vi "数据查询.vi"() -> ()   [LabVIEW 2014]
uses:
  <vilib>/Analysis/baseanly.llb/Mean (DBL).vi
  <vilib>/Analysis/NI_AALBase.lvlib
panel:
  out "平均温度: 2":dbl caption="平均温度:"
  out "最低温度: 2":dbl caption="最低温度:"
  out "最高温度: 2":dbl caption="最高温度:"
  in  "返回":bool
  in  "导出报表":bool
  in  "高级查询":bool
  in  "查询":bool
  in  "查询结果":i32(listbox)
  in  "结束时间：":timestamp format="%<%y/%m/%d>T"
  in  "开始时间：":timestamp format="%<%y/%m/%d>T"
  out "平均温度:":dbl
  out "最低温度:":dbl
  out "最高温度:":dbl
  out "温度":cluster{sgl, sgl}[](graph)
  # "数据查询起止时间设置"
  # "采集参数"
  # "进口温度"
  # "出口温度"
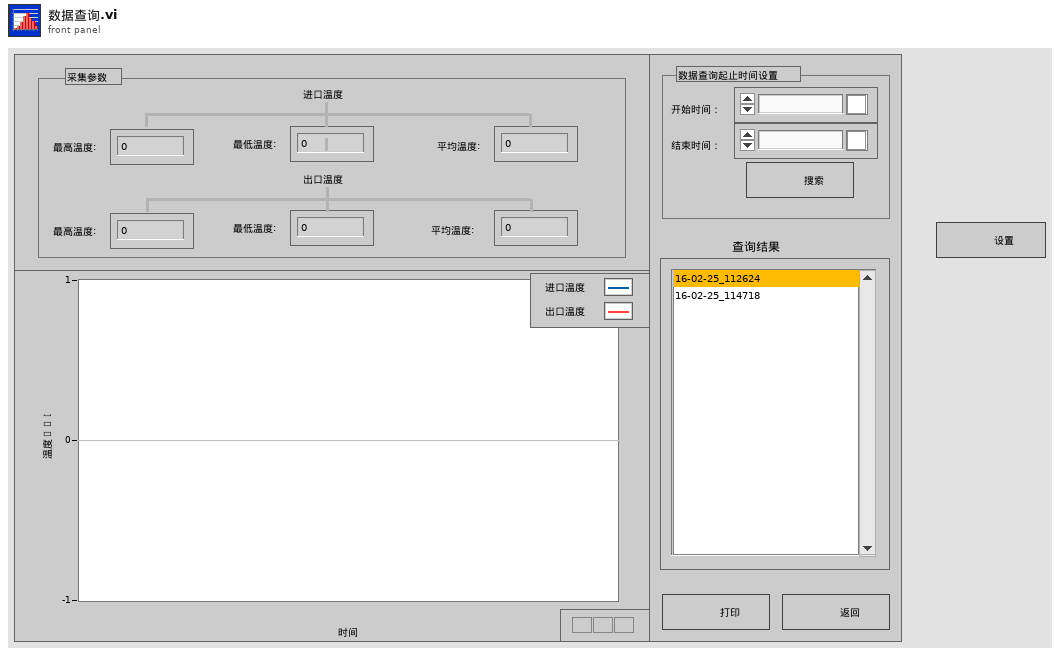
[diagram p1: front panel]
types:
  T1 = enum16{"open", "open or create", "create or replace", "create", "open (read-only)"}
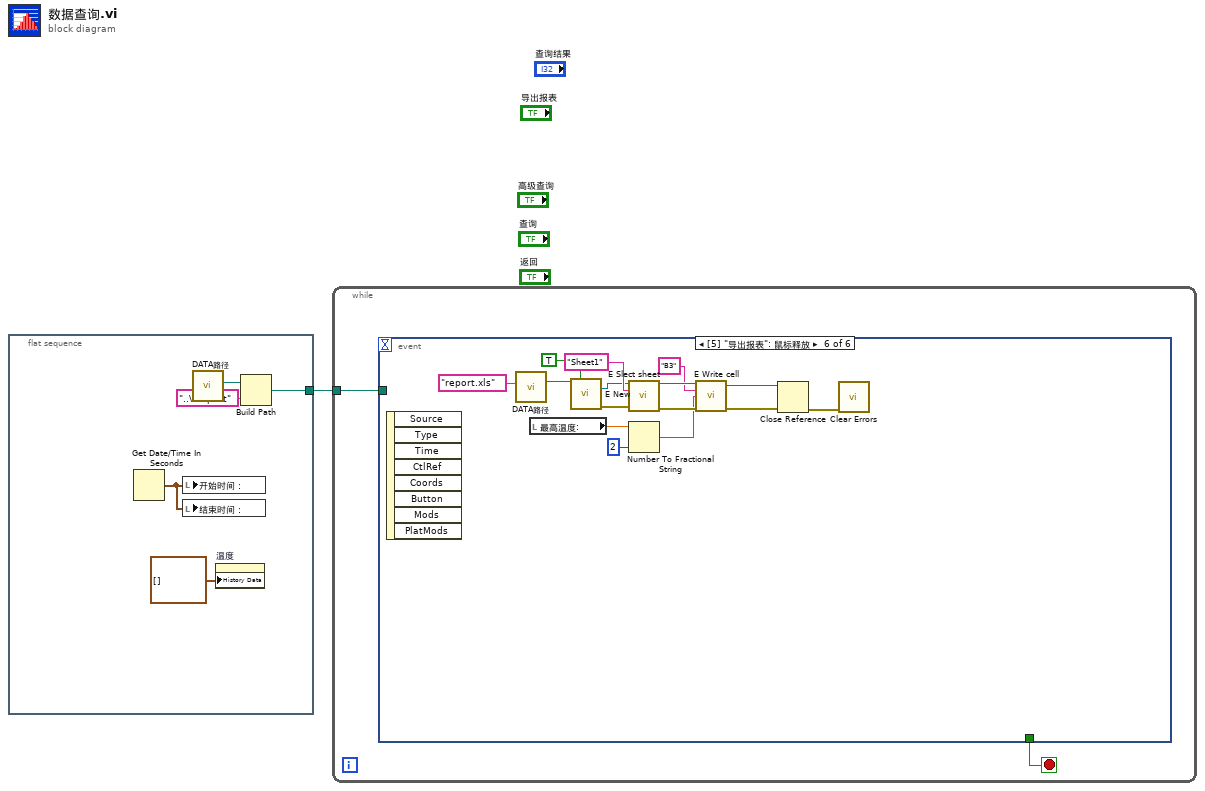
[diagram p0: block diagram]
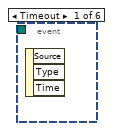
[diagram p2: hidden frame]
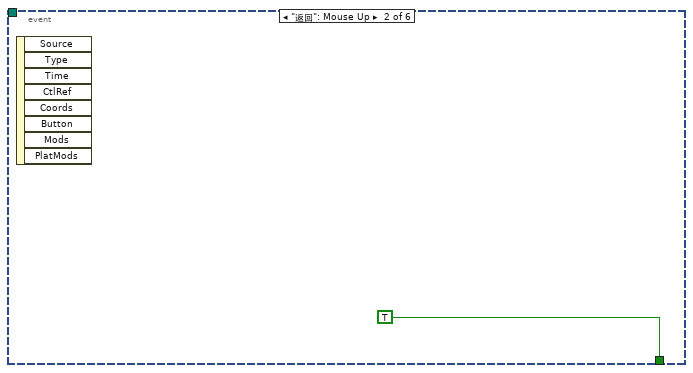
[diagram p3: hidden frame]
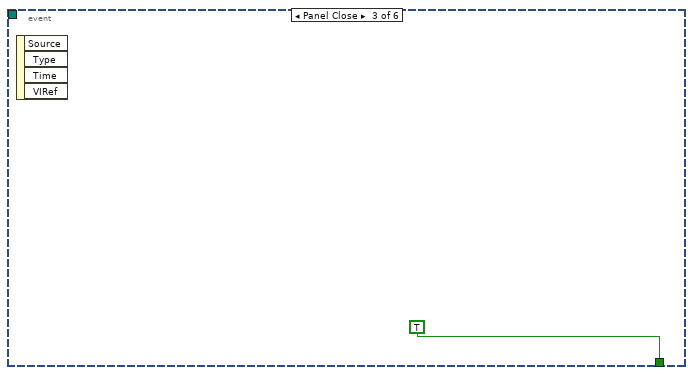
[diagram p4: hidden frame]
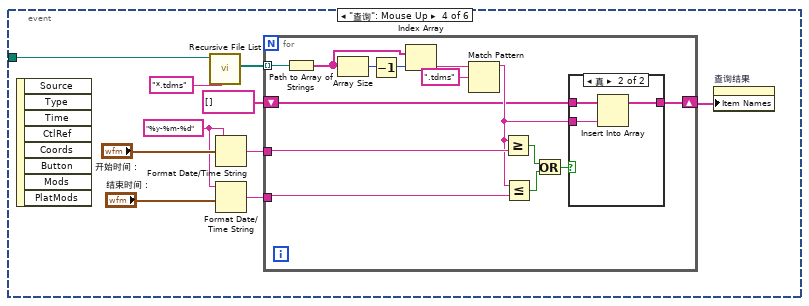
[diagram p5: hidden frame]
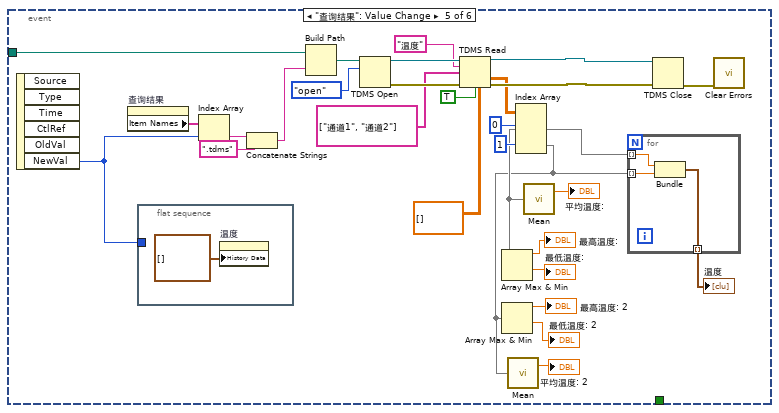
[diagram p7: hidden frame]
diagram:
  n1 = flat-sequence {
    tunnel: [w4] -> w1
    frame #0 {
      n2 = Get Date/Time In Seconds() -> (seconds since 1Jan1904=w3:timestamp)
      n3 = local write "开始时间："(w3) -> ()
      n4 = local write "结束时间："(w3) -> ()
      n5 = call "DATA路径.vi"() -> ("DATA路径"=w6:path)  [unwired: 11 in]
      n6 = property on="温度" class="WFChart (严格)"("History Data"=cluster{sgl, sgl}[] [] ("历史数据")) -> ()  [unwired: 2 in, 2 out]
      n7 = Build Path(base path=w6, name or relative path="..\\Report" ("名称或相对路径")) -> (appended path=w4:path)
    }
  }
  n8 = while {
    tunnel: w1 -> [w7]
    stop <- w8 stop-if-true
    n9 = event shown="[5] \"导出报表\": 鼠标释放" {
      selector: _ -> [_ _ _ _ _ _]
      dyn-events: _ -> [_ _ _ _ _ _]
      timeout: _ -> [_ _ _ _ _ _]
      tunnel: [_ TRUE TRUE _ _ _] -> w8
      tunnel: w7 -> [_ _ _ w17 w66 _]
      event Timeout {
        n10 = event-data() -> ()  [unwired: 1 in, 3 out]
      }
      event "返回": Mouse Up {
        n11 = event-data() -> ()  [unwired: 1 in, 8 out]
      }
      event Panel Close {
        n12 = event-data() -> ()  [unwired: 1 in, 4 out]
      }
      event "查询": Mouse Up {
        w18 = "%y-%m-%d" ("时间格式字符串(%c)")
        n13 = event-data() -> ()  [unwired: 1 in, 8 out]
        n14 = call <vilib>:"Recursive File List.vi"("pattern"="*.tdms", "Folder Path"=w17) -> ("All Files in Dir"=w15:path[])  [unwired: 5 in, 4 out]
        n15 = Format Date/Time String(time format string (%c)=w18, seconds (now)="开始时间：") -> (date/time string=w14:string)  [unwired: 1 in]
        n16 = Format Date/Time String(time format string (%c)=w18, seconds (now)="结束时间：") -> (date/time string=w13:string)  [unwired: 1 in]
        n17 = for {
          tunnel: w15 -> [w34] mode=indexing
          tunnel: w14 -> [w28]
          tunnel: w13 -> [w27]
          shift-right: [w22] -> w11
          shift-left: string[] [] -> [w21]
          n18 = Path to Array of Strings(0:w34) -> (2:w31:string[])  [unwired: 1 out]
          n19 = Array Size(array=w31) -> (size(s)=w33:i32)
          n20 = Decrement(x=w33) -> (x-1=w32:i32)
          n21 = Index Array(array=w31, index=w32) -> (element=w30:string)
          n22 = Match Pattern(string=w30, regular expression=".tdms" ("正则表达式")) -> (before substring=w23:string)  [unwired: 1 in, 3 out]
          n23 = Greater Or Equal?(x=w23, y=w28) -> (x >= y?=w25:bool)
          n24 = Less Or Equal?(x=w23, y=w27) -> (x <= y?=w24:bool)
          n25 = Or(x=w25, y=w24) -> (x .or. y?=w26:bool)
          n26 = case shown="真" w26 {
            tunnel: w23 -> [_ w38]
            tunnel: [w35 w37] -> w22
            tunnel: w21 -> [w35 w36]
            frame False {
            }
            frame True {
              n27 = Insert Into Array(array=w36, new element=w38) -> (w37:string[])  [unwired: 1 in]
            }
          }
        }
        n28 = property on="查询结果" class="LstBox (严格)"("Item Names"=w11) -> ()  [unwired: 2 in, 2 out]
      }
      event "查询结果": Value Change {
        n29 = event-data() -> ("NewVal"=w47:i32)  [unwired: 1 in, 5 out]
        n30 = property on="查询结果" class="LstBox (严格)"() -> ("Item Names"=w67:string[])  [unwired: 2 in, 2 out]
        n31 = flat-sequence {
          tunnel: w47 -> [_]
          frame #0 {
            n32 = property on="温度" class="WFChart (严格)"("History Data"=cluster{sgl, sgl}[] [] ("历史数据")) -> ()  [unwired: 2 in, 2 out]
          }
        }
        n33 = Index Array(array=w67, index=w47) -> (element=w65:string)
        n34 = Concatenate Strings(w65, ".tdms" ("字符串")) -> (w63:string)
        n35 = Build Path(base path=w66, name or relative path=w63) -> (appended path=w62:path)
        n36 = TDMS Open(10:T1."open" ("操作(0:open)"), 11:w62) -> (0:w59:errorcluster, 3:w60:refnum<k34>)  [unwired: 5 in]
        n37 = TDMS Read(0:w60, 5:"温度" ("组名称输入"), 7:string[] ["通道1", "通道2"] ("通道名输入（无标题）"), 11:w59, 12:sgl[][] [] ("添加的数组"), 13:TRUE ("按文件顺序返回通道？(F)")) -> (4:w56:refnum<k34>, 10:w52:sgl[][], 15:w55:errorcluster)  [unwired: 2 in, 3 out]
        n38 = Index Array(array=w52, index (row) #1=0 ("索引 (行)"), index (row) #2=1 ("索引 (行)")) -> (element #1=w42:sgl[], element #2=w39:sgl[])  [unwired: 2 in]
        n39 = Array Max & Min(array=w42) -> (max value=→"最高温度:":sgl, min value=→"最低温度:":sgl)  [unwired: 2 out]
        n40 = Array Max & Min(array=w39) -> (max value=→"最高温度: 2":sgl, min value=→"最低温度: 2":sgl)  [unwired: 2 out]
        n41 = call-poly <vilib>:"Mean.vi"("X"=w39) -> ("mean"=→"平均温度: 2":dbl)  [unwired: 1 out]
        n42 = call-poly <vilib>:"Mean.vi"("X"=w42) -> ("mean"=→"平均温度:":dbl)  [unwired: 1 out]
        n43 = for {
          tunnel: w42 -> [w71] mode=indexing
          tunnel: [w70] -> w53 mode=indexing
          tunnel: w39 -> [w69] mode=indexing
          n44 = Bundle(w71, w69) -> (w70:cluster{sgl, sgl})  [unwired: 1 in]
        }
        "温度" <- w53
        n45 = TDMS Close(8:w55, 11:w56) -> (0:w57:errorcluster)  [unwired: 1 out]
        n46 = call <vilib>:"Clear Errors.vi"("error in (no error)"=w57) -> ()  [unwired: 5 in, 2 out]
      }
      event "导出报表": Mouse Up {
        n47 = event-data() -> ()  [unwired: 1 in, 8 out]
        n48 = call "DATA路径.vi"("文件名"="report.xls") -> ("DATA路径"=w85:path)  [unwired: 10 in]
        n49 = local read "最高温度:"() -> (w75:dbl)
        n50 = call "E New.vi"("model Path/模板路径"=w85, "Visible/表格可见？(False)"=TRUE) -> ("Excel._Workbook"=w72:refnum<k7>, "Error Out"=w84:errorcluster)  [unwired: 11 in, 1 out]
        n51 = call "E Slect sheet.vi"("Excel._Workbook"=w72, "Sheet Name/工作表名称(Sheet1)"="Sheet1", "error in (no error)"=w84) -> ("Excel._Worksheet"=w82:refnum<k7>, "error out"=w81:errorcluster)  [unwired: 11 in]
        n52 = Number To Fractional String(number=w75, precision (6)=i16 2 ("精度(6)")) -> (F-format string=w73:string)  [unwired: 2 in]
        n53 = call "E Write cell.vi"("Excel._Worksheet"=w82, "Cell/表格位置"="B3", "data/数据"=w73, "error in (no error)"=w81) -> ("Excel._Worksheet"=w79:refnum<k7>, "error out"=w78:errorcluster)  [unwired: 9 in, 1 out]
        n54 = Close Reference(reference=w79, error in (no error)=w78) -> (error out=w77:errorcluster)
        n55 = call <vilib>:"Clear Errors.vi"("error in (no error)"=w77) -> ()  [unwired: 5 in, 2 out]
      }
    }
  }
